vi "NI OCR-Initialize.vi"(8 "error in":errorcluster, 11 "VI Refnum":refnum<vi>) -> (0 "error out":errorcluster, 3 "Buffer Data":T1={"VI Refnum"=refnum, "Src Image"=refnum, "Dst Image"=refnum, "Ctl Refnum []"=[], "Ctl Label"=[], "User Event"=refnum, "Event Registration Refnum"=refnum, "Timeout"=0, "IMAQ OCR Session"=refnum, "Objects"=[], "ROI Descriptor"={"Global Rectangle"=[], "Contours"=[]}, "Settings"={"Objects"=0, "Threshold"=128, "Reject Border"=FALSE, "Fill Holes"=FALSE, "Min Object Size"=FALSE, "Min Size"=3, "Max Object Size"=FALSE, "Max Size"=100, "Show Search Area"=FALSE, "Show Center"=TRUE, "Show Bounding Box"=TRUE}} {"Settings"."Objects" items=["Bright Objects", "Dark Objects"]; "Settings"."Threshold" min=1 max=999999999 step=1; "Settings"."Max Size" min=1 max=999999999 step=1; "Settings"."Min Size" min=1 max=999999999 step=1; "ROI Descriptor"."Contours"."Type" items=["No Selection", "Point", "Line", "Rectangle", "Oval", "Polygon", "Freehand Region", "Annulus", "Unused2", "Unused3", "Broken Line", "Freehand Line", "Rotated Rectangle"]; "Objects"."Aspect Ratio" format="%.2f"; "Objects"."Orientation" format="%.2f"; "Objects"."Area" format="%.2f"; "Objects"."Object Center"."Y" format="%.2f"; "Objects"."Object Center"."X" format="%.2f"})   [LabVIEW 2016]
uses:
  Data Def/NI OCR-Buffer Data.ctl
  <vilib>/vision/Image Controls.llb/IMAQ Image.ctl
  Data Def/NI OCR-User Event Data.ctl
  <vilib>/vision/OCR.llb/IMAQ OCR Session.ctl
  <vilib>/Utility/miscctls.llb/LVPointTypeDef.ctl
  <vilib>/vision/NI_Vision_Development_Module.lvlib
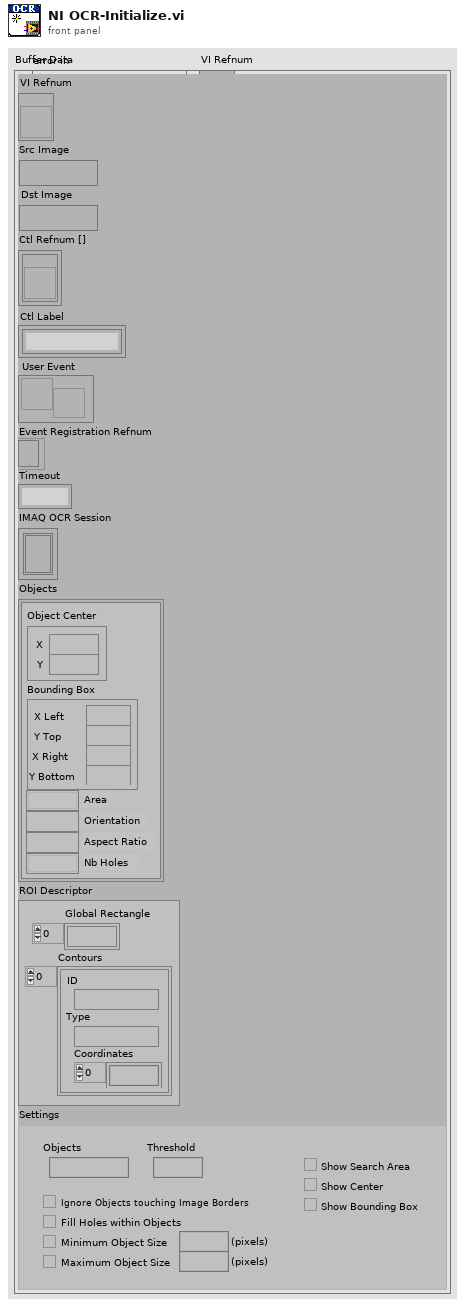
[diagram p1: front panel]
types:
  T1 = typedef "NI OCR-Buffer Data.ctl" = cluster{"VI Refnum":refnum<vi>, "Src Image":T2, "Dst Image":T2, "Ctl Refnum []":refnum<vi>[], "Ctl Label":string[], "User Event":refnum<user-event>, "Event Registration Refnum":refnum<event-registration>, "Timeout":i32, "IMAQ OCR Session":T3, "Objects":cluster{"Object Center":cluster{"X":sgl, "Y":sgl}, "Bounding Box":cluster{"X Left":i32, "Y Top":i32, "X Right":i32, "Y Bottom":i32}, "Area":sgl, "Orientation":sgl, "Aspect Ratio":sgl, "Nb Holes":i32}[], "ROI Descriptor":T4, "Settings":cluster{"Objects":u16, "Threshold":i32, "Reject Border":bool, "Fill Holes":bool, "Min Object Size":bool, "Min Size":i32, "Max Object Size":bool, "Max Size":i32, "Show Search Area":bool, "Show Center":bool, "Show Bounding Box":bool}}
  T2 = typedef "IMAQ Image.ctl" = refnum<image>
  T3 = typedef "IMAQ OCR Session.ctl" = refnum<k1>
  T4 = typedef "ROI Descriptor" = cluster{"Global Rectangle":i32[], "Contours":cluster{"ID":enum32{"External", "Internal"}, "Type":u32, "Coordinates":i32[]}[]}
  T5 = typedef "LVPointTypeDef.ctl" = cluster{"Horizontal":i16, "Vertical":i16}
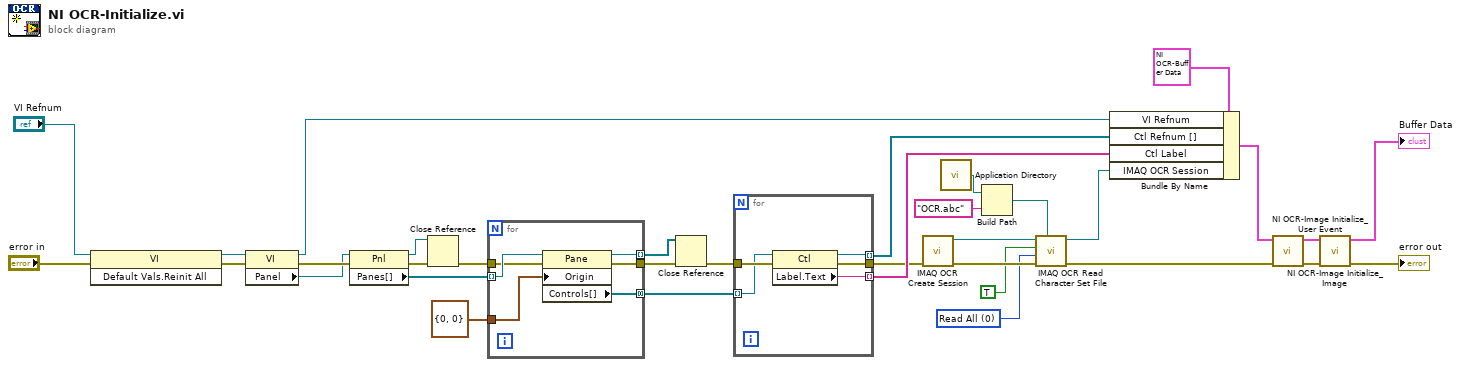
[diagram p0: block diagram]
diagram:
  w1 = 0 items=["Read All", "Read Character Set Only", "Read Properties Only"] ("Read Options")
  n1 = invoke class="VI" method="Default Vals.Reinit All"(reference="VI Refnum", error in="error in") -> (reference out=w31:refnum<vi>, error out=w32:errorcluster)  [unwired: 1 in, 1 out]
  n2 = property class="VI"(reference=w31, error in=w32) -> (reference out=w18:refnum<vi>, error out=w30:errorcluster, "Panel"=w29:refnum<vi>)
  n3 = property class="Pnl"(reference=w29, error in=w30) -> (reference out=w25:refnum<vi>, error out=w26:errorcluster, "Panes[]"=w28:refnum<vi>[])
  n4 = Close Reference(reference=w25, error in (no error)=w26) -> (error out=w24:errorcluster)
  n5 = for {
    tunnel: w24 -> [w39]
    tunnel: w28 -> [w40] mode=indexing
    tunnel: T5 {"Horizontal"=0, "Vertical"=0} ("Origin") -> [w38]
    tunnel: [w37] -> w21 mode=concatenating
    tunnel: [w36] -> w23
    tunnel: [w35] -> w22 mode=indexing
    n6 = property class="Pane"(reference=w40, error in=w39, "Origin"=w38) -> (reference out=w35:refnum<vi>, error out=w36:errorcluster, "Controls[]"=w37:refnum<vi>[])
  }
  n7 = Close Reference(reference=w22, error in (no error)=w23) -> (error out=w20:errorcluster)
  n8 = for {
    tunnel: w21 -> [w44] mode=indexing
    tunnel: w20 -> [w45]
    tunnel: [w43] -> w10
    tunnel: [w42] -> w16 mode=indexing
    tunnel: [w41] -> w17 mode=indexing
    n9 = property class="Ctl"(reference=w44, error in=w45) -> (reference out=w41:refnum<vi>, error out=w43:errorcluster, "Label.Text"=w42:string)
  }
  n10 = call "IMAQ OCR Create Session"("error in (no error)"=w10) -> ("error out"=w9:errorcluster, "IMAQ OCR Session"=w8:T3)  [unwired: 9 in]
  n11 = call <vilib>:"Application Directory.vi"() -> ("Application Directory"=w4:path)
  n12 = Build Path(base path=w4, name or relative path="OCR.abc") -> (appended path=w3:path)
  n13 = call "IMAQ OCR Read Character Set File"("File Path"=w3, "error in (no error)"=w9, "Read Options"=w1, "Append To Character Set? (F)"=TRUE, "IMAQ OCR Session"=w8) -> ("error out"=w7:errorcluster, "IMAQ OCR Session (dup)"=w6:T3)  [unwired: 4 in, 1 out]
  n14 = Bundle By Name(cluster=T1 {"VI Refnum"=refnum, "Src Image"=refnum, "Dst Image"=refnum, "Ctl Refnum []"=[], "Ctl Label"=[], "User Event"=refnum, "Event Registration Refnum"=refnum, "Timeout"=-1, "IMAQ OCR Session"=refnum, "Objects"=[], "ROI Descriptor"={"Global Rectangle"=[], "Contours"=[]}, "Settings"={"Objects"=0, "Threshold"=128, "Reject Border"=FALSE, "Fill Holes"=FALSE, "Min Object Size"=FALSE, "Min Size"=3, "Max Object Size"=FALSE, "Max Size"=100, "Show Search Area"=FALSE, "Show Center"=TRUE, "Show Bounding Box"=TRUE}} ("Buffer Data"), "VI Refnum"=w18, "Ctl Refnum []"=w17, "Ctl Label"=w16, "IMAQ OCR Session"=w6) -> (w15:T1)
  n15 = call "NI OCR-Image Initialize_User Event.vi"("error in"=w7, "Buffer Data In"=w15) -> ("error out"=w14:errorcluster, "Buffer Data Out"=w13:T1)  [unwired: 8 in]
  n16 = call "NI OCR-Image Initialize_Image.vi"("error in"=w14, "Buffer Data In"=w13) -> ("error out"=→"error out":errorcluster, "Buffer Data Out"=→"Buffer Data":T1)  [unwired: 8 in]
